vi "Shooting Logic.vi"(8 "Shoot Override?":bool, 9 "Ready to Fire?":bool, 10 "In Range?":bool, 11 "is gunner ready to shoot?":bool) -> (3 "Shooting":bool)   [LabVIEW 2019, in "Robot.lvlib" / "Panzer.lvclass"]
uses:
  Panzer.lvclass
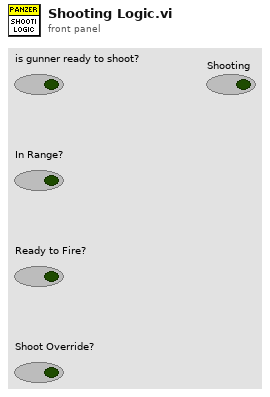
[diagram p1: front panel]
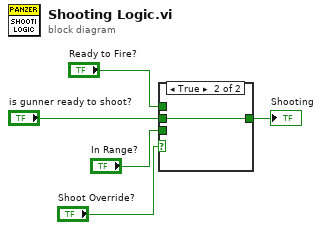
[diagram p0: block diagram]
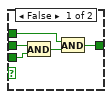
[diagram p2: hidden frame]
diagram:
  n1 = case shown="True" "Shoot Override?" {
    tunnel: "is gunner ready to shoot?" -> [w10 w11]
    tunnel: "In Range?" -> [w9 _]
    tunnel: "Ready to Fire?" -> [w8 _]
    tunnel: [w6 w11] -> w2
    frame False {
      n2 = And(x=w10, y=w9) -> (x .and. y?=w7:bool)
      n3 = And(x=w8, y=w7) -> (x .and. y?=w6:bool)
    }
    frame True {
    }
  }
  "Shooting" <- w2
